vi "Add Or Replace History Array.vi"(0 "History XY Buffer In":T1(array[cluster]), 1 "History XY In":T2(array[cluster]), 2 "Index":i32, 4 "# of points":i32) -> (7 "History XY Buffer Out":T1(array[cluster]))   [LabVIEW 2013]
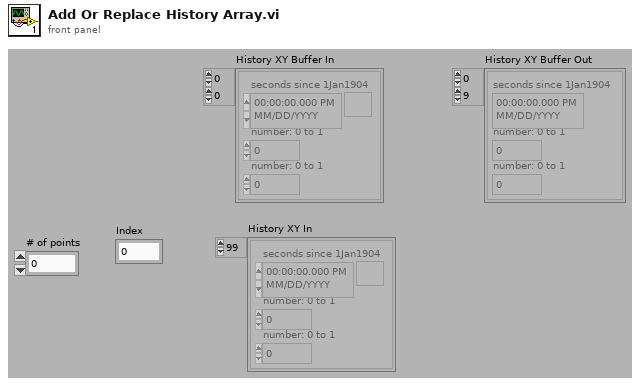
[diagram p1: front panel]
types:
  T1 = cluster{"seconds since 1Jan1904":timestamp, "number: 0 to 1":dbl, "number: 0 to 1":dbl}[][]
  T2 = cluster{"seconds since 1Jan1904":timestamp, "number: 0 to 1":dbl, "number: 0 to 1":dbl}[]
  T3 = cluster{"seconds since 1Jan1904":timestamp, "number: 0 to 1":dbl, "number: 0 to 1":dbl}
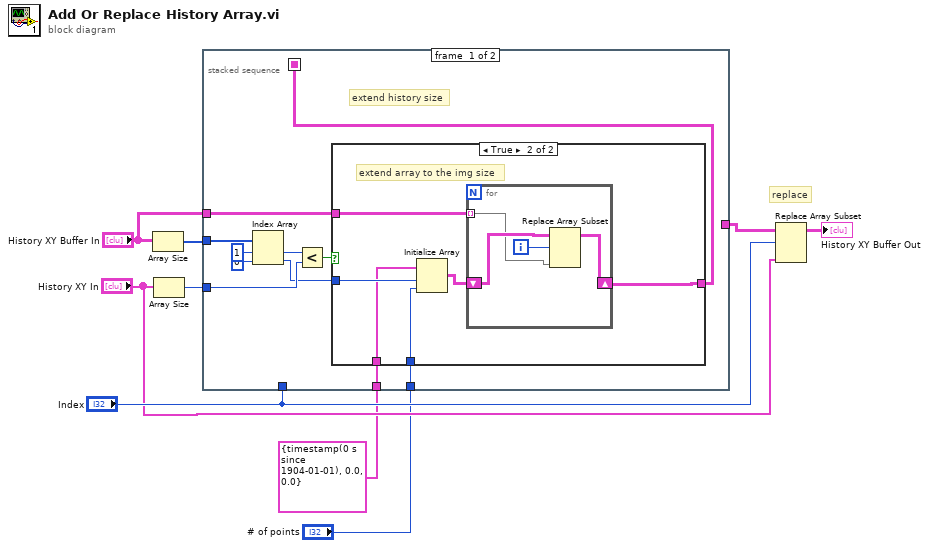
[diagram p0: block diagram]
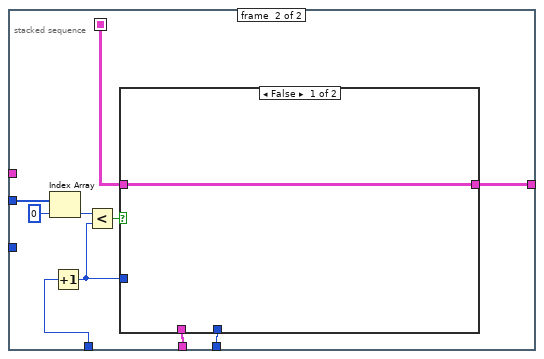
[diagram p3: hidden frame]
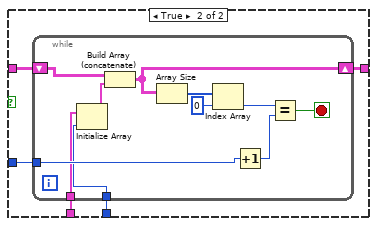
[diagram p4: hidden frame]
diagram:
  # "replace"
  n1 = Array Size(array="History XY Buffer In") -> (size(s)=w8:i32[])
  n2 = Array Size(array="History XY In") -> (size(s)=w7:i32)
  n3 = stacked-sequence {
    seq-local: [w18 _] -> [_ w38]
    tunnel: [_ w41] -> w6
    tunnel: "Index" -> [_ w35]
    tunnel: w8 -> [w16 w37]
    tunnel: w7 -> [w17 _]
    tunnel: "History XY Buffer In" -> [w14 _]
    tunnel: T3 {"seconds since 1Jan1904"=timestamp(0 s since 1904-01-01), "number: 0 to 1"=0.0, "number: 0 to 1"=0.0} -> [w11 w34]
    tunnel: "# of points" -> [w10 w33]
    frame #0 {
      # "extend history size"
      n4 = Index Array(array=w16, index #1=1 ("length"), index #2=0 ("index")) -> (element #1=w15:i32, element #2=w12:i32)
      n5 = Less?(x=w15, y=w17) -> (x < y?=w19:bool)
      n6 = case shown="True" w19 {
        tunnel: [w21 w27] -> w18
        tunnel: w14 -> [w21 w26]
        tunnel: w12 -> [_ w25]
        tunnel: w11 -> [_ w24]
        tunnel: w10 -> [_ w23]
        frame False {
        }
        frame True {
          # "extend array to the img size"
          n7 = Initialize Array(w24, w25, w23) -> (w22:T1)
          n8 = for {
            tunnel: w26 -> [w28] mode=indexing
            shift-right: [w30] -> w27
            shift-left: w22 -> [w29]
            i -> [w31]
            n9 = Replace Array Subset(array=w29, new element=w28, index (row)=w31) -> (w30:T1)  [unwired: 1 in]
          }
        }
      }
    }
    frame #1 {
      n10 = Index Array(array=w37, index=0) -> (element=w36:i32)
      n11 = Increment(x=w35) -> (x+1=w32:i32)
      n12 = Less?(x=w36, y=w32) -> (x < y?=w39:bool)
      n13 = case shown="False" w39 {
        tunnel: [w42 w47] -> w41
        tunnel: w38 -> [w42 w46]
        tunnel: w32 -> [_ w45]
        tunnel: w34 -> [_ w44]
        tunnel: w33 -> [_ w43]
        frame False {
        }
        frame True {
          n14 = while {
            shift-right: [w58] -> w47
            shift-left: w46 -> [w52]
            tunnel: w45 -> [w51]
            tunnel: w44 -> [w49]
            tunnel: w43 -> [w48]
            stop <- w57 stop-if-true
            n15 = Initialize Array(w49, w48) -> (w50:T2)
            n16 = Build Array (concatenate)(w52, w50) -> (w58:T1)
            n17 = Array Size(array=w58) -> (size(s)=w54:i32[])
            n18 = Index Array(array=w54, index=0) -> (element=w53:i32)
            n19 = Increment(x=w51) -> (x+1=w56:i32)
            n20 = Equal?(x=w53, y=w56) -> (x = y?=w57:bool)
          }
        }
      }
    }
  }
  n21 = Replace Array Subset(array=w6, new element="History XY In", index (row)="Index") -> (→"History XY Buffer Out":T1)  [unwired: 1 in]
